vi "GET_Statistics_(offline).vi"(6 "Error In":errorcluster, 8 "Histogram parameters":T2={"max"=300.0, "min"=0.0, "# bins"=10, "threshold"=0.0, "thr. type"=enum."higher accepted"}, 9 "Data vector in":dbl[](array[numeric])) -> (0 "Error Out":errorcluster, 1 "Mean thresholded":dbl, 2 "Perc. thresholded":dbl, 3 "Histogram data out":T1)   [LabVIEW 2018, in "Tracker.lvlib"]
uses:
  Tracker.lvlib
  Controls/CTL_Histogram_parameters.ctl
  <vilib>/Analysis/baseanly.llb/Mean (DBL).vi
  <vilib>/Analysis/NI_AALPro.lvlib
  <vilib>/Analysis/NI_AALBase.lvlib
  Common_Resources.lvlib
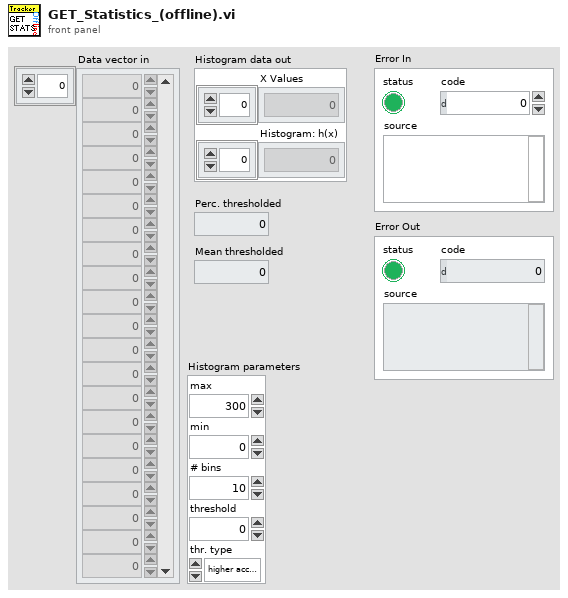
[diagram p1: front panel]
types:
  T1 = cluster{"X Values":dbl[], "Histogram: h(x)":dbl[]}
  T2 = typedef "Common_Resources.lvlib/CTL_Histogram_parameters.ctl" = cluster{"max":dbl, "min":dbl, "# bins":i32, "threshold":dbl, "thr. type":enum16{"higher accepted", "lower accepted"}}
  T3 = cluster{"X Values":dbl[], "Histogram: h(x)":i32[]}
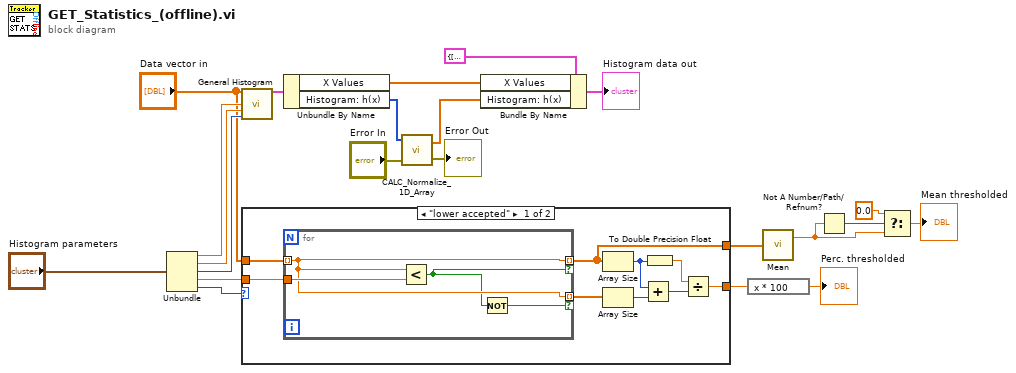
[diagram p0: block diagram]
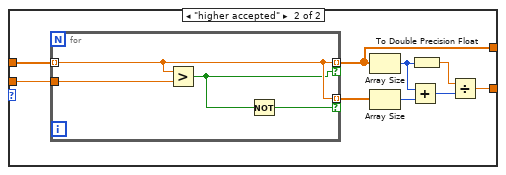
[diagram p2: hidden frame]
diagram:
  n1 = Unbundle("Histogram parameters") -> ("max"=w16:dbl, "min"=w15:dbl, "# bins"=w14:i32, "threshold"=w8:dbl, "thr. type"=w9:enum16{"higher accepted", "lower accepted"})
  n2 = call <vilib>:"General Histogram.vi"("X"="Data vector in", "max"=w16, "min"=w15, "# bins"=w14) -> ("Histogram Graph"=w21:T3)  [unwired: 7 in, 4 out]
  n3 = case shown="\"lower accepted\"" w9 {
    tunnel: "Data vector in" -> [w31 w44]
    tunnel: w8 -> [w30 w43]
    tunnel: [w24 w37] -> w7
    tunnel: [w23 w36] -> w5
    frame "lower accepted" {
      n4 = for {
        tunnel: w31 -> [w34] mode=indexing
        tunnel: w30 -> [w35]
        tunnel: [w34] -> w23 mode=indexing if=w33
        tunnel: [w34] -> w29 mode=indexing if=w32
        n5 = Less?(x=w34, y=w35) -> (x < y?=w33:bool)
        n6 = Not(x=w33) -> (.not. x?=w32:bool)
      }
      n7 = Array Size(array=w23) -> (size(s)=w27:i32)
      n8 = Array Size(array=w29) -> (size(s)=w28:i32)
      n9 = Add(x=w27, y=w28) -> (x+y=w26:i32)
      n10 = To Double Precision Float(number=w27) -> (double precision float=w25:dbl)
      n11 = Divide(x=w25, y=w26) -> (x/y=w24:dbl)
    }
    frame "higher accepted" {
      n12 = for {
        tunnel: w44 -> [w47] mode=indexing
        tunnel: w43 -> [w48]
        tunnel: [w47] -> w36 mode=indexing if=w46
        tunnel: [w47] -> w42 mode=indexing if=w45
        n13 = Greater?(x=w47, y=w48) -> (0:w46:bool)
        n14 = Not(x=w46) -> (.not. x?=w45:bool)
      }
      n15 = Array Size(array=w36) -> (size(s)=w40:i32)
      n16 = Array Size(array=w42) -> (size(s)=w41:i32)
      n17 = Add(x=w40, y=w41) -> (x+y=w39:i32)
      n18 = To Double Precision Float(number=w40) -> (double precision float=w38:dbl)
      n19 = Divide(x=w38, y=w39) -> (x/y=w37:dbl)
    }
  }
  n20 = Unbundle By Name(w21) -> ("X Values"=w18:dbl[], "Histogram: h(x)"=w22:i32[])
  n21 = call "CALC_Normalize_1D_Array.vi"("Error In"="Error In", "1D array"=w22) -> ("Error Out"=→"Error Out":errorcluster, "Normalized 1D array"=w19:dbl[])  [unwired: 1 in]
  n22 = Bundle By Name(cluster=T1 {"X Values"=[15.0, 45.0, 75.0, 105.0, 135.0, 165.0, 195.0, 225.0, 255.0, 285.0], "Histogram: h(x)"=[-1.0, -1.0, 0.0, 1.0, 2.0, 1.0, 0.0, -1.0, -1.0, -1.0]} ("XY Graph - Light"), "X Values"=w18, "Histogram: h(x)"=w19) -> (→"Histogram data out":T1)
  n23 = expression code="x * 100"(w7) -> (→"Perc. thresholded":dbl)
  n24 = call-poly <vilib>:"Mean.vi"("X"=w5) -> ("mean"=w2:dbl)  [unwired: 1 out]
  n25 = Not A Number/Path/Refnum?(number/path/refnum=w2) -> (NaN/Path/Refnum?=w4:bool)
  n26 = Select(t=0.0, s=w4, f=w2) -> (s? t:f=→"Mean thresholded":dbl)
